vi "Create.vi"(8 "error in (no error)":errorcluster, 10 "Subsystem Name (optional)":string, 11 "SMO":refnum<class "SMO.lvclass">) -> (0 "error out":errorcluster, 2 "SMO name":string, 3 "SMO out":refnum<class "SMO.lvclass">)   [LabVIEW 2013, in "SMO.lvclass"]
doc: "Constructor\n\nNote 01: This method is overridable by descendant\nNote 02: When overridden, Call Parent Method is required\n\n---------------------------------------------------------------\nJKI State Machine Objects™\nhttp://jki.net/state-machine-objects/\nCopyright (C) 2005-2015, JKI <info@jki.net>\nALL RIGHTS RESERVED"
uses:
  SMO.lvclass
  SMO.lvclass/SMO.ctl
  Typedefs/Process Error Notification--Cluster.ctl
  Typedefs/SMOState --Enum.ctl
  Registry/Registry-SMO.lvclass
panel:
  # "For instructions on how to use the JKI State Machine Objects, examples and video tutorials, visit:\nhttp://jki.net/state-machine-objects/\n\nJKI State Machine Objects™\nhttp://jki.net/state-machine-objects/\nCopyright (C) 2005-2015, JKI <info@jki.net>\nALL RIGHTS RESERVED"
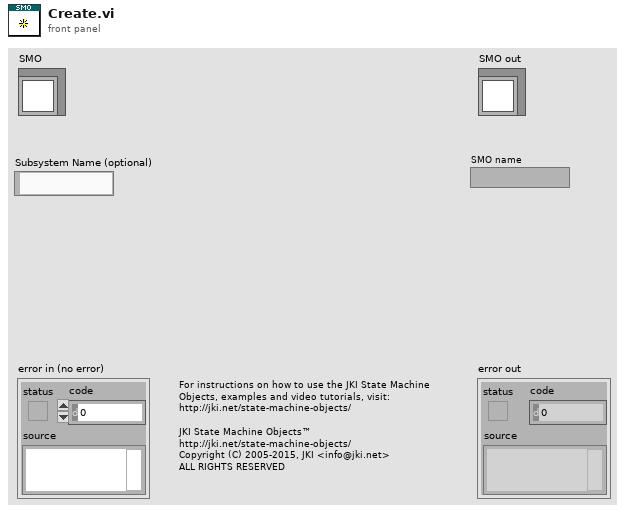
[diagram p1: front panel]
types:
  T1 = typedef "SMO.lvclass/SMOState --Enum.ctl" = enum16{"unknown", "Created", "Started", "Stopped"}
  T2 = typedef "SMO.lvclass/Process Error Notification--Cluster.ctl" = cluster{"error":errorcluster}
  T3 = typedef "SMO.lvclass/PrivateData--Ref.ctl" = refnum<data-value>
  T4 = typedef "SMO.lvclass/PrivateData--Cluster.ctl" = cluster{"Parent Call":T5, "Registered Processes":T6[], "Sync Notifier":refnum<notifier>, "Process Error Notifier":refnum<notifier>, "Protected Events":T7, "Public Events":T8, "SMO State":T1, "[Dependencies]":T9[], "[Attributes]":refnum<class "Attribute.lvclass">[], "Launcher Close":refnum<notifier>}
  T5 = typedef "SMO.lvclass/Parent Call--Enum.ctl" = enum16{"Allows parent to run", "Does not request parent to run"}
  T6 = typedef "SMO.lvclass/RegisteredProcessData--Cluster.ctl" = cluster{"Name":string, "Static VI Ref":refnum<vi>, "Running":bool, "NotifierRef":u32}
  T7 = typedef "SMO.lvclass/Protected Events.ctl" = cluster{"StopProcesses":refnum<user-event>, "AbortProcesses":refnum<user-event>, "Config Changed":refnum<user-event>}
  T8 = typedef "SMO.lvclass/Public Events.ctl" = cluster{"Error":refnum<user-event>, "State":refnum<user-event>}
  T9 = typedef "SMO.lvclass/SMO Dependency--Cluster.ctl" = cluster{"Dependency":refnum<class "SMO.lvclass">, "Level":string}
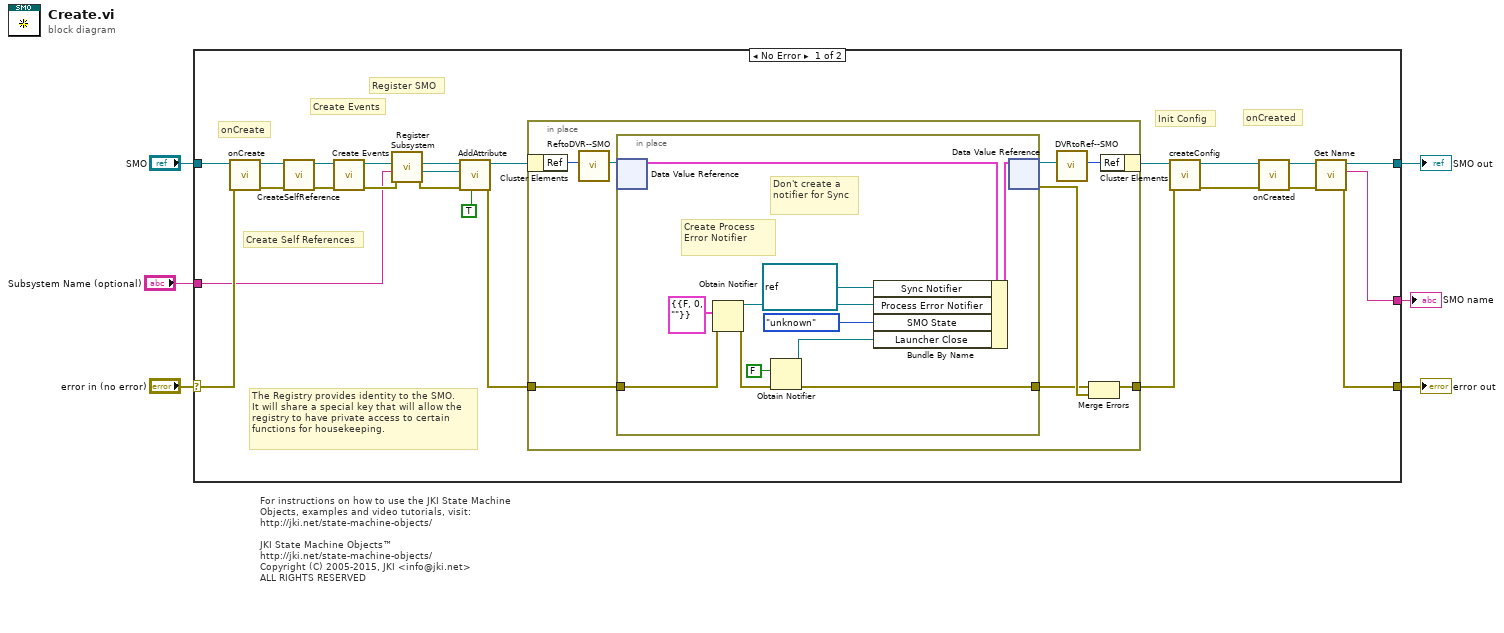
[diagram p0: block diagram]
diagram:
  # "For instructions on how to use the JKI State Machine Objects, examples and video tutorials, visit:\nhttp://jki.net/state-machine-objects/\n\nJKI State Machine Objects™\nhttp://jki.net/state-machine-objects/\nCopyright (C) 2005-2015, JKI <info@jki.net>\nALL RIGHTS RESERVED"
  n1 = case shown="No Error" "error in (no error)" {
    selector: "error in (no error)" -> [w27 w51]
    tunnel: [w22 w51] -> w5
    tunnel: [w24 w50] -> w3
    tunnel: "SMO" -> [w28 w50]
    tunnel: "Subsystem Name (optional)" -> [w26 _]
    tunnel: [w21 _] -> w1
    frame No Error {
      # "Init Config"
      # "The Registry provides identity to the SMO.\nIt will share a special key that will allow the\nregistry to have private access to certain\nfunctions for housekeeping."
      # "Create Self References"
      # "onCreated"
      # "Register SMO"
      # "Create Events"
      # "onCreate"
      n2 = call-dynamic "onCreate.vi"("error in (no error)"=w27, "SMO"=w28) -> ("error out"=w14:errorcluster, "SMO out"=w16:refnum<class "SMO.lvclass">)  [unwired: 8 in]
      n3 = call-dynamic "CreateSelfReference.vi"("error in (no error)"=w14, "SMO"=w16) -> ("error out"=w13:errorcluster, "SMO out"=w15:refnum<class "SMO.lvclass">)  [unwired: 8 in]
      n4 = call "Create Events.vi"("error in (no error)"=w13, "SMO"=w15) -> ("error out"=w29:errorcluster, "SMO out"=w30:refnum<class "SMO.lvclass">)  [unwired: 8 in]
      n5 = call "Register Subsystem.vi"("error in (no error)"=w29, "Subsystem Name (optional)"=w26, "JKI SMO in"=w30) -> ("error out"=w18:errorcluster, "Attribute.Identity"=w12:refnum<class "Attribute.Identity.lvclass">, "JKI SMO out"=w20:refnum<class "SMO.lvclass">)  [unwired: 6 in]
      n6 = call "AddAttribute.vi"("Overwrite? (F)"=TRUE, "error in (no error)"=w18, "Attribute"=w12, "SMO in"=w20) -> ("error out"=w17:errorcluster, "SMO out"=w19:refnum<class "SMO.lvclass">)  [unwired: 6 in]
      n7 = in-place {
        in-place-border: [w37] -> w7
        in-place-border: w17 -> [w35]
        n8 = in-place-cluster #1(w19) -> ("Ref"=w34:u32)
        n9 = call "ReftoDVR--SMO.vi"("Ref"=w34) -> ("Ref"=w33:T3)  [unwired: 10 in]
        n10 = in-place {
          in-place-border: [w40] -> w36
          in-place-border: w35 -> [w45]
          # "Don't create a notifier for Sync"
          # "Create Process Error Notifier"
          n11 = in-place-dvr #2(w33) -> (w49:T4)  [unwired: 1 out]
          n12 = Obtain Notifier(notification data type=T2 {"error"={"status"=FALSE, "code"=0, "source"=""}} ("Process Notification"), error in (no error)=w45) -> (notifier out=w47:refnum<notifier>, error out=w41:errorcluster)  [unwired: 2 in, 1 out]
          n13 = Obtain Notifier(notification data type=FALSE ("Launcher Close"), error in (no error)=w41) -> (notifier out=w39:refnum<notifier>, error out=w40:errorcluster)  [unwired: 2 in, 1 out]
          n14 = Bundle By Name(cluster=w49, "Sync Notifier"=refnum<notifier> refnum, "Process Error Notifier"=w47, "SMO State"=SMOState_--Enum."unknown", "Launcher Close"=w39) -> (w48:T4)
          n15 = in-place-dvr #2(w48) -> (w32:T3, w38:errorcluster)
        }
        n16 = call "DVRtoRef--SMO.vi"("Ref"=w32) -> ("Ref"=w31:u32)  [unwired: 10 in]
        n17 = Merge Errors(w36, w38) -> (w37:errorcluster)
        n18 = in-place-cluster #1("Ref"=w31) -> (w10:refnum<class "SMO.lvclass">)
      }
      n19 = call "createConfig.vi"("error in (no error)"=w7, "SMO in"=w10) -> ("error out"=w8:errorcluster, "SMO out"=w9:refnum<class "SMO.lvclass">)  [unwired: 8 in]
      n20 = call-dynamic "onCreated.vi"("error in (no error)"=w8, "SMO"=w9) -> ("error out"=w23:errorcluster, "SMO out"=w25:refnum<class "SMO.lvclass">)  [unwired: 8 in]
      n21 = call "Get Name.vi"("error in (no error)"=w23, "SMO"=w25) -> ("error out"=w22:errorcluster, "Name"=w21:string, "SMO out"=w24:refnum<class "SMO.lvclass">)  [unwired: 7 in]
    }
    frame Error {
    }
  }
  "error out" <- w5
  "SMO out" <- w3
  "SMO name" <- w1
